vi "8gainunpack.vi"(0 "GAIN & CHANNEL SELECTOR":T1={"0"=1, "1"=1, "2"=1, "3"=1, "4"=1, "5"=1, "6"=1, "7"=1}, 1 "Monopolar":bool) -> (2 "Number of channels":i32, 3 "channels (0)":i32[](array[numeric]), 4 "Input Limits":cluster{"High Limit":dbl, "Low Limit":dbl}[](array[cluster]) {"High Limit" format="%.3f"; "Low Limit" format="%.3g"})   [LabVIEW 2025]
doc: "Unpacks a cluster of 8 gains creating a channel and gain vector by skipping over those channels with 0 gain. Creates an array of scaling factors. Also outputs the number of active channels.\nScott Hannahs, FBNML, Jan 1992\nAuthor: Scott Hannahs <sth@magnet.fsu.edu>\n\nThis software is licensed for use under the “MIT License\"\nCopyright (c) 2025 Scott Hannahs, sth@sth@magnet.sthnet.net\n\nPermission is hereby granted, free of charge, to any person obtaining a copy of this software and associated documentation files (the \"Software\"), to deal in the Software without restriction, including without limitation the rights to use, copy, modify, merge, publish, distribute, sublicense, and/or sell copies of the Software, and to permit persons to whom the Software is furnished to do so, subject to the following conditions: The above copyright notice and this permission notice shall be included in all copies or substantial portions of the Software.\n\nTHE SOFTWARE IS PROVIDED \"AS IS\", WITHOUT WARRANTY OF ANY KIND, EXPRESS OR IMPLIED, INCLUDING BUT NOT LIMITED TO THE WARRANTIES OF MERCHANTABILITY, FITNESS FOR A PARTICULAR PURPOSE AND NONINFRINGEMENT. IN NO EVENT SHALL THE AUTHORS OR COPYRIGHT HOLDERS BE LIABLE FOR ANY CLAIM, DAMAGES OR OTHER LIABILITY, WHETHER IN AN ACTION OF CONTRACT, TORT OR OTHERWISE, ARISING FROM, OUT OF OR IN CONNECTION WITH THE SOFTWARE OR THE USE OR OTHER DEALINGS IN THE SOFTWARE."
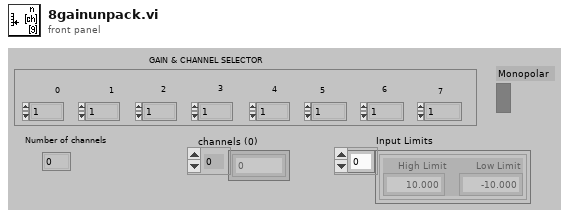
[diagram p1: front panel]
types:
  T1 = cluster{"0":i16, "1":i16, "2":i16, "3":i16, "4":i16, "5":i16, "6":i16, "7":i16}
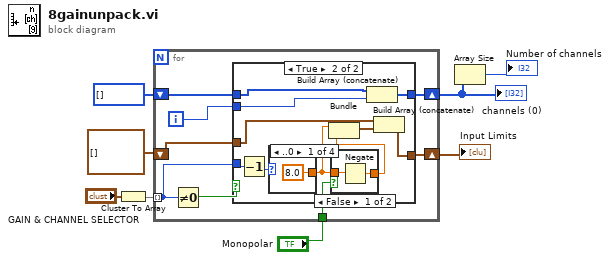
[diagram p0: block diagram]
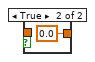
[diagram p3: hidden frame]
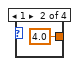
[diagram p4: hidden frame]
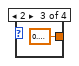
[diagram p5: hidden frame]
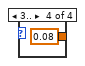
[diagram p6: hidden frame]
diagram:
  n1 = Cluster To Array(cluster="GAIN & CHANNEL SELECTOR") -> (array=w7:i16[])
  n2 = for {
    shift-right: [w12] -> w3
    shift-left: i32[] [] -> [w9]
    shift-right: [w16] -> w4
    shift-left: cluster{sgl, sgl}[] [] -> [w15]
    tunnel: w7 -> [w14] mode=indexing
    tunnel: "Monopolar" -> [w11]
    i -> [w10]
    n3 = Not Equal To 0?(x=w14) -> (x != 0?=w13:bool)
    n4 = case shown="True" w13 {
      tunnel: w15 -> [w18 w27]
      tunnel: w14 -> [_ w28]
      tunnel: [w17 w26] -> w12
      tunnel: [w18 w29] -> w16
      tunnel: w11 -> [_ w21]
      tunnel: w10 -> [_ w20]
      tunnel: w9 -> [w17 w19]
      frame False {
      }
      frame True {
        n5 = Decrement(x=w28) -> (x-1=w25:i16)
        n6 = case shown="..0" w25 {
          tunnel: [8.0 sgl 4.0 sgl 0.8 0.08] -> w23
          frame ..0 {
          }
          frame 1 {
          }
          frame 2 {
          }
          frame 3.. {
          }
        }
        n7 = case shown="False" w21 {
          tunnel: w23 -> [w31 _]
          tunnel: [w30 0.0] -> w24
          frame False {
            n8 = Negate(x=w31) -> (-x=w30:dbl)
          }
          frame True {
          }
        }
        n9 = Bundle(w23, w24) -> (w22:cluster{dbl, dbl})  [unwired: 1 in]
        n10 = Build Array (concatenate)(w19, w20) -> (w26:i32[])
        n11 = Build Array (concatenate)(w27, w22) -> (w29:cluster{dbl, dbl}[])
      }
    }
  }
  "Input Limits" <- w4
  "channels (0)" <- w3
  n12 = Array Size(array=w3) -> (size(s)=→"Number of channels":i32)
